vi "save_presets.vi"(8 "error in (no error)":errorcluster, 11 "ColorOverlay in":refnum<class "ColorOverlay.lvclass">) -> (0 "error out":errorcluster, 3 "ColorOverlay out":refnum<class "ColorOverlay.lvclass">)   [LabVIEW 2010, in "ColorOverlay.lvclass"]
uses:
  ColorOverlay.lvclass
  presets_save_cluster.ctl
  cursor_cluster.ctl
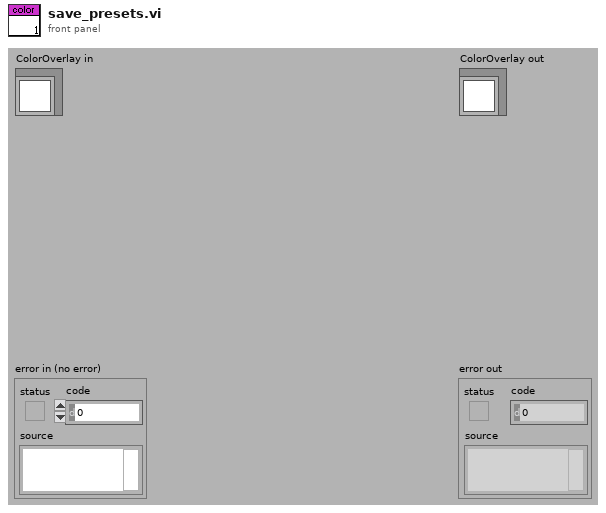
[diagram p1: front panel]
types:
  T1 = typedef "ColorOverlay.lvclass/presets_save_cluster.ctl" = cluster{"# hot pixels":i32, "# cold pixels":i32, "color lower limit":u32, "color upper limit":u32, "color?":bool, "start color":u8[], "end color":u8[], "array of cursors":T2[]}
  T2 = typedef "ColorOverlay.lvclass/cursor_cluster.ctl" = cluster{"cursor position":dbl[]}
  T3 = typedef "ColorOverlay.lvclass/settings_cluster.ctl" = cluster{"# cold pixels":i32, "# hot pixels":i32, "graph editor":cluster{"ramp array out":u32[]}[], "color lower limit":u32, "color upper limit":u32, "color?":bool, "start color":cluster{u8, u8, u8, u8}, "end color":cluster{u8, u8, u8, u8}, "array of cursors":T2[]}
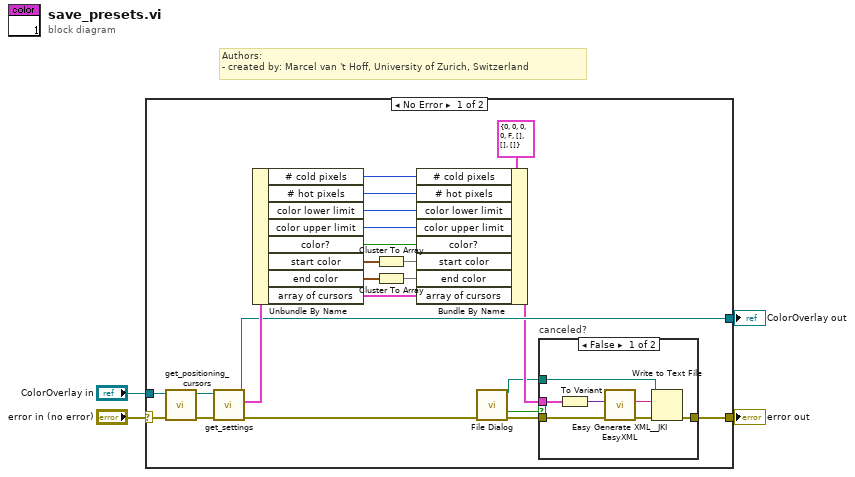
[diagram p0: block diagram]
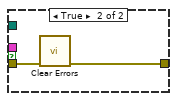
[diagram p2: hidden frame]
diagram:
  # "Authors: \n- created by: Marcel van 't Hoff, University of Zurich, Switzerland"
  n1 = case shown="No Error" "error in (no error)" {
    selector: "error in (no error)" -> [w17 w38]
    tunnel: [w13 w38] -> w3
    tunnel: [w15 w37] -> w1
    tunnel: "ColorOverlay in" -> [w27 w37]
    frame No Error {
      n2 = call-dynamic "get_positioning_cursors.vi"("error in (no error)"=w17, "ColorOverlay in"=w27) -> ("error out"=w26:errorcluster, "ColorOverlay out"=w16:refnum<class "ColorOverlay.lvclass">)  [unwired: 8 in]
      n3 = call-dynamic "get_settings.vi"("error in (no error)"=w26, "ColorOverlay in"=w16) -> ("error out"=w12:errorcluster, "settings cluster"=w25:T3, "ColorOverlay out"=w15:refnum<class "ColorOverlay.lvclass">)  [unwired: 7 in]
      n4 = Unbundle By Name(w25) -> ("# cold pixels"=w23:i32, "# hot pixels"=w22:i32, "color lower limit"=w21:u32, "color upper limit"=w20:u32, "color?"=w19:bool, "start color"=w8:cluster{u8, u8, u8, u8}, "end color"=w6:cluster{u8, u8, u8, u8}, "array of cursors"=w18:T2[])
      n5 = Cluster To Array(cluster=w8) -> (array=w7:u8[])
      n6 = Cluster To Array(cluster=w6) -> (array=w5:u8[])
      n7 = Bundle By Name(cluster=T1 {"# hot pixels"=0, "# cold pixels"=0, "color lower limit"=0, "color upper limit"=0, "color?"=FALSE, "start color"=[], "end color"=[], "array of cursors"=[]} ("presets save cluster"), "# cold pixels"=w23, "# hot pixels"=w22, "color lower limit"=w21, "color upper limit"=w20, "color?"=w19, "start color"=w7, "end color"=w5, "array of cursors"=w18) -> (w14:T1)
      n8 = call "File Dialog"("error in"=w12) -> ("selected path"=w10:path, "cancelled"=w9:bool, "error out"=w11:errorcluster)  [unwired: 11 in, 1 out]
      n9 = case "canceled?" shown="False" w9 {
        tunnel: w14 -> [w34 _]
        tunnel: [w31 w35] -> w13
        tunnel: w11 -> [w32 w36]
        tunnel: w10 -> [w29 _]
        frame False {
          n10 = To Variant(anything=w34) -> (Variant=w28:variant)
          n11 = call <vilib>:"Easy Generate XML__JKI EasyXML.vi"("error in (no error)"=w32, "LabVIEW Data"=w28) -> ("error out"=w33:errorcluster, "XML String"=w30:string)  [unwired: 8 in]
          n12 = Write to Text File(file (use dialog)=w29, text=w30, error in=w33) -> (error out=w31:errorcluster)  [unwired: 1 in, 2 out]
        }
        frame True {
          n13 = call <vilib>:"Clear Errors.vi"("error in (no error)"=w36) -> ("error out"=w35:errorcluster)  [unwired: 6 in]
        }
      }
    }
    frame Error {
    }
  }
  "error out" <- w3
  "ColorOverlay out" <- w1
